vi "ViewHistory.vi"(11 "file path":path) -> ()   [LabVIEW 2020]
uses:
  <vilib>/Utility/miscctls.llb/LVAnnotationListTypeDef.ctl
panel:
  in  "拟合通道":u16(ring) caption="拟合通道：" items=["电流1", "电流1反应性", "电流2", "电流2反应性", "棒位D", "棒位C", "电压6"]
  in  "拟合按钮":bool
  in  "另存数据":bool
  in  "同步数据":bool
  out "历史波形图":cluster{dbl, dbl, dbl[][]}(graph)
  # "坐标轴与图例"
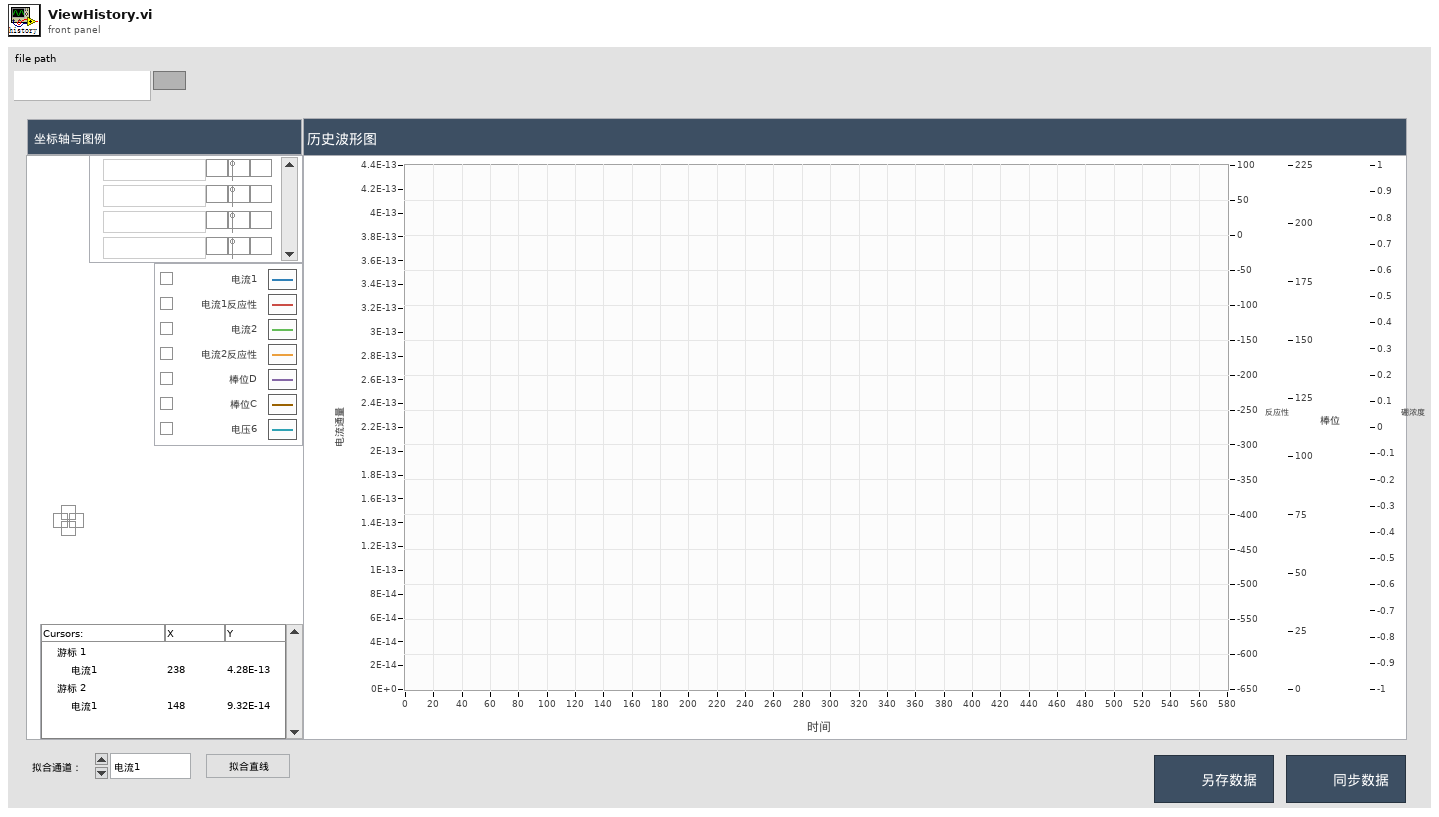
[diagram p1: front panel]
types:
  T1 = typedef "LVAnnotationListTypeDef.ctl" = cluster{"Name":string, "Color":u32, "Style":u8, "Point Style":u8, "Name Visible":bool, "Allow Drag":bool, "Annotation Mode":u32, "Plot":i32, "Index":i32, "Position":cluster{"X":dbl, "Y":dbl}, "X Scale":u32, "Y Scale":u32, "Show Arrow":bool, "Lock Name":bool, "Plot Area":i32, "Label Offset":cluster{"X":dbl, "Y":dbl}}[]
  T2 = cluster{"Name":string, "Color":u32, "Style":u8, "Point Style":u8, "Name Visible":bool, "Allow Drag":bool, "Annotation Mode":u32, "Plot":i32, "Index":i32, "Position":cluster{"X":dbl, "Y":dbl}, "X Scale":u32, "Y Scale":u32, "Show Arrow":bool, "Lock Name":bool, "Plot Area":i32, "Label Offset":cluster{"X":dbl, "Y":dbl}}
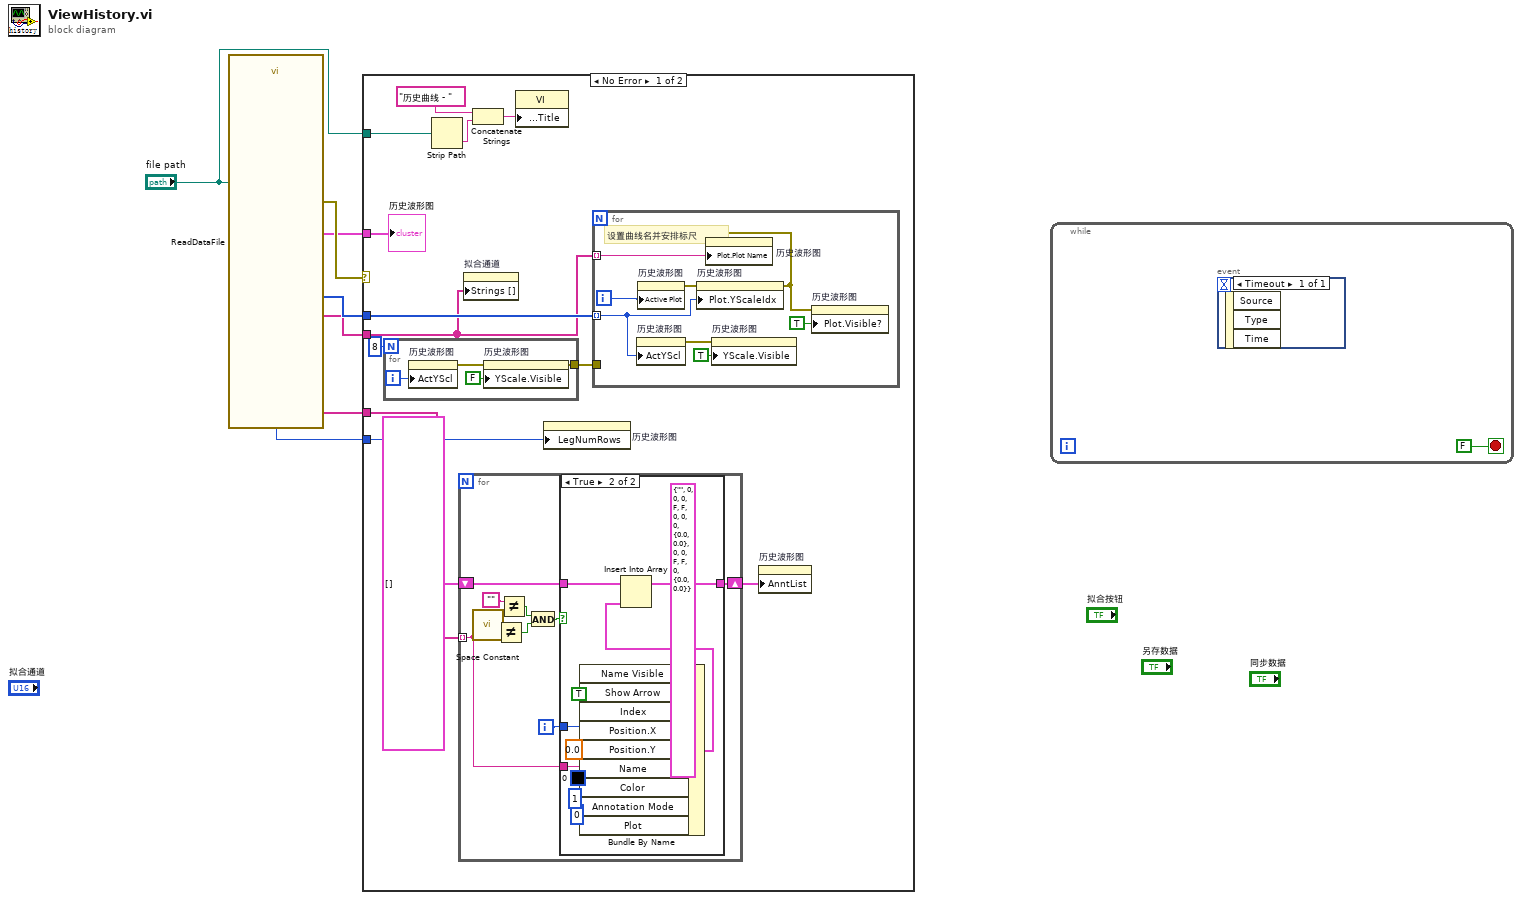
[diagram p0: block diagram]
diagram:
  n1 = call "ReadDataFile.vi"("file path"="file path") -> ("曲线对应标尺编号"=w3:i32[], "曲线名"=w2:string[], "曲线数"=w5:i32, "error out"=w7:errorcluster, "备注数组"=w4:string[], "波形簇"=w6:cluster{dbl, dbl, dbl[][]})  [unwired: 2 in, 7 out]
  n2 = case shown="No Error" w7 {
    tunnel: w6 -> [w20 _]
    tunnel: w5 -> [w19 _]
    tunnel: w4 -> [w16 _]
    tunnel: w3 -> [w15 _]
    tunnel: w2 -> [w8 _]
    tunnel: "file path" -> [w11 _]
    frame No Error {
      n3 = for {
        N: 8 -> [_]
        tunnel: [w21] -> w10
        i -> [w22]
        n4 = property on="历史波形图" class="WFGraph (strict)"("ActYScl"=w22) -> (error out=w24:errorcluster)  [unwired: 2 in, 1 out]
        n5 = property on="历史波形图" class="WFGraph (strict)"(error in=w24, "YScale.Visible"=FALSE ("Y Scale.Visible")) -> (error out=w21:errorcluster)  [unwired: 1 in, 1 out]
      }
      n6 = Strip Path(path=w11) -> (name=w12:string)  [unwired: 1 out]
      n7 = for {
        tunnel: w16 -> [w36] mode=indexing
        shift-right: [w38] -> w18
        shift-left: T1 [] ("注释列表") -> [w39]
        i -> [w40]
        n8 = call <vilib>:"Space Constant.vi"() -> ("String"=w41:string)
        n9 = Not Equal?(x=w41, y=w36) -> (x != y?=w34:bool)
        n10 = Not Equal?(x="", y=w36) -> (x != y?=w35:bool)
        n11 = And(x=w35, y=w34) -> (x .and. y?=w33:bool)
        n12 = case shown="True" w33 {
          tunnel: w36 -> [_ w48]
          tunnel: w40 -> [_ w50]
          tunnel: w39 -> [w42 w53]
          tunnel: [w42 w52] -> w38
          frame False {
          }
          frame True {
            w51 = TRUE ("Show Arrow")
            n13 = Bundle By Name(cluster=T2 {"Name"="", "Color"=0, "Style"=0, "Point Style"=0, "Name Visible"=FALSE, "Allow Drag"=FALSE, "Annotation Mode"=0, "Plot"=0, "Index"=0, "Position"={"X"=0.0, "Y"=0.0}, "X Scale"=0, "Y Scale"=0, "Show Arrow"=FALSE, "Lock Name"=FALSE, "Plot Area"=0, "Label Offset"={"X"=0.0, "Y"=0.0}} ("元素"), "Name Visible"=w51, "Show Arrow"=w51, "Index"=w50, "Position.X"=w50, "Position.Y"=0.0 ("Y"), "Name"=w48, "Color"=u32 0, "Annotation Mode"=u32 1, "Plot"=0) -> (w49:T2)
            n14 = Insert Into Array(array=w53, new element=w49) -> (w52:T1)  [unwired: 1 in]
          }
        }
      }
      n15 = property on="拟合通道" class="Ring (strict)"("Strings []"=w8) -> ()  [unwired: 2 in, 2 out]
      n16 = Concatenate Strings("历史曲线 - " ("string"), w12) -> (w13:string)
      n17 = property class="VI"("Front Panel.Title"=w13) -> ()  [unwired: 2 in, 2 out]
      n18 = property on="历史波形图" class="WFGraph (strict)"("LegNumRows"=w19) -> ()  [unwired: 2 in, 2 out]
      n19 = for {
        tunnel: w15 -> [w28] mode=indexing
        tunnel: w8 -> [w30] mode=indexing
        tunnel: w10 -> [_]
        i -> [w31]
        # "设置曲线名并安排标尺"
        n20 = property on="历史波形图" class="WFGraph (strict)"("ActYScl"=w28) -> (error out=w29:errorcluster)  [unwired: 2 in, 1 out]
        n21 = property on="历史波形图" class="WFGraph (strict)"("Active Plot"=w31) -> (error out=w32:errorcluster)  [unwired: 2 in, 1 out]
        n22 = property on="历史波形图" class="WFGraph (strict)"(error in=w32, "Plot.YScaleIdx"=w28) -> (error out=w25:errorcluster)  [unwired: 1 in, 1 out]
        n23 = property on="历史波形图" class="WFGraph (strict)"(error in=w25, "Plot.Plot Name"=w30) -> ()  [unwired: 1 in, 2 out]
        n24 = property on="历史波形图" class="WFGraph (strict)"(error in=w29, "YScale.Visible"=TRUE ("Y Scale.Visible")) -> ()  [unwired: 1 in, 2 out]
        n25 = property on="历史波形图" class="WFGraph (strict)"(error in=w25, "Plot.Visible?"=TRUE ("Y Scale.Visible")) -> ()  [unwired: 1 in, 2 out]
      }
      n26 = property on="历史波形图" class="WFGraph (strict)"("AnntList"=w18) -> ()  [unwired: 2 in, 2 out]
      "历史波形图" <- w20
    }
    frame Error {
    }
  }
  n27 = while {
    stop <- FALSE stop-if-true
    n28 = event shown="[0] Timeout" {
      selector: _ -> [_]
      dyn-events: _ -> [_]
      timeout: _ -> [_]
      event Timeout {
        n29 = event-data() -> ()  [unwired: 1 in, 3 out]
      }
    }
  }
